vi "AccessData.vi"(0 "Sensitivity1":i32=1, 1 "Sensitivity2":i32=1, 2 "Sensitivity3":i32=1, 3 "Sensitivity4":i32=1, 4 "输入簇":T2, 6 "CH1Enable":bool, 8 "CH2Enable":bool, 10 "CH3Enable":bool, 12 "CH4Enable":bool, 13 "RmOffset":bool, 14 "SamplRate1":T1(ring)=enum."105.468", 15 "SamplRate2":T1(ring)=enum."105.468", 16 "SamplRate3":T1(ring)=enum."105.468", 17 "SamplRate4":T1(ring)=enum."105.468") -> (7 "VibrationWave":dbl[][](array[numeric]) caption="数组", 9 "Speed":u16[](array[numeric]), 11 "Error":bool, 18 "输出簇":T2)   [LabVIEW 2012]
uses:
  <vilib>/measure/madcrms.llb/Basic Averaged DC-RMS for 1 Chan.vi
  <vilib>/measure/NI_MAPro.lvlib
panel:
  out "Humidity_Channel":u8
  out "Temperature_Channel7":u8
  out "Temperature_Channel6":dbl
  out "Temperature_Channel5":dbl
  out "Temperature_Channel4":dbl
  out "Temperature_Channel3":dbl
  out "Temperature_Channel2":dbl
  out "Temperature_Channel1":dbl
  out "系统时间":string
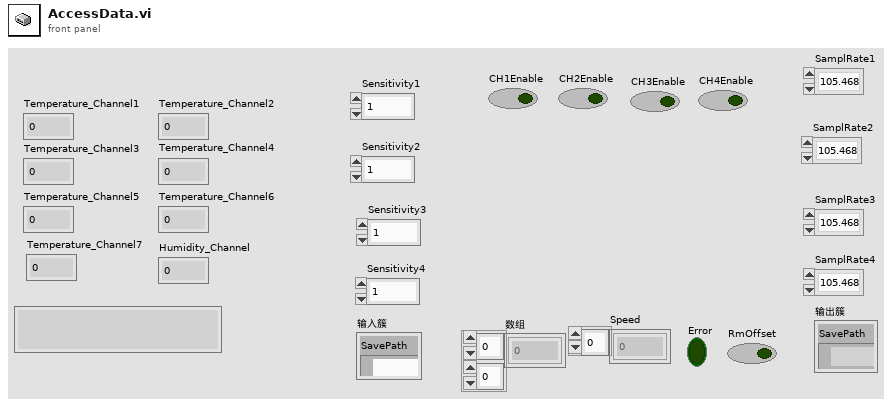
[diagram p1: front panel]
types:
  T1 = enum16{"", "105.468", "52.734", "35.156", "26.367", "21.094", "17.578", "15.067", "13.184", "11.719", "10.545"}
  T2 = cluster{"SavePath":path, "SAVE?":bool, "connection ID":refnum<k5>}
  T3 = enum16{"open", "replace", "create", "open or create", "replace or create", "replace or create with confirmation"}
  T4 = enum16{"big-endian, network order", "native, host order", "little-endian"}
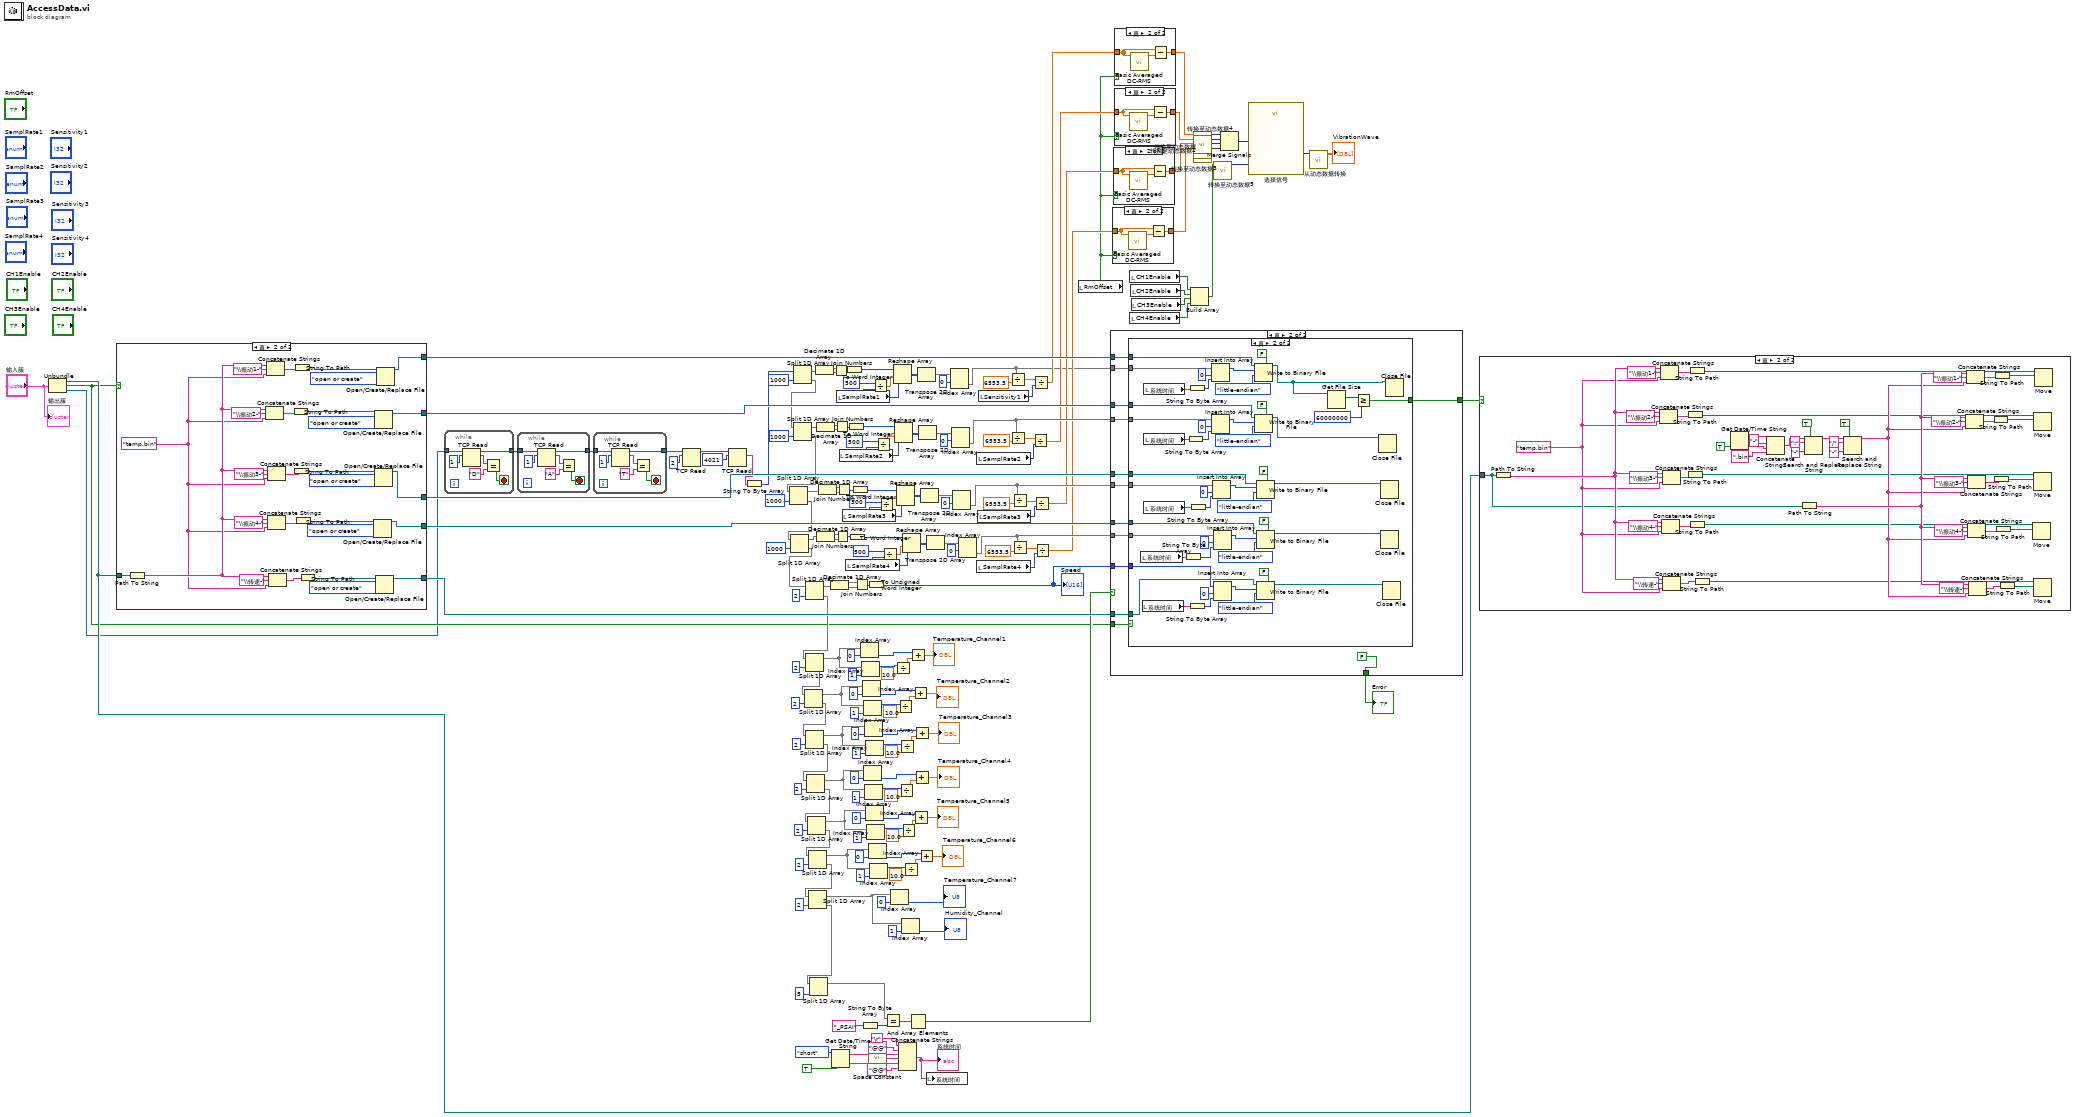
[diagram p0: block diagram]
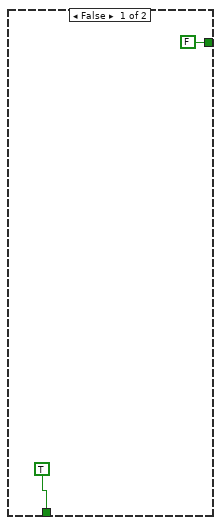
[diagram p6: hidden frame]
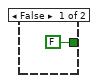
[diagram p7: hidden frame]
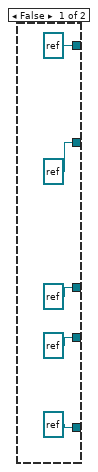
[diagram p8: hidden frame]
diagram:
  n1 = Unbundle("输入簇") -> ("SavePath"=w31:path, "SAVE?"=w30:bool, "connection ID"=w29:refnum<k5>)
  n2 = case shown="真" w30 {
    tunnel: [refnum<file> refnum ("refnum out") w231] -> w198
    tunnel: [refnum<file> refnum ("refnum out") w230] -> w197
    tunnel: [refnum<file> refnum ("refnum out") w229] -> w196
    tunnel: [refnum<file> refnum ("refnum out") w228] -> w195
    tunnel: [refnum<file> refnum ("refnum out") w227] -> w194
    tunnel: w31 -> [_ w204]
    frame False {
    }
    frame True {
      w205 = "temp.bin" ("字符串")
      n3 = Path To String(path=w204) -> (string=w211:string)
      n4 = Concatenate Strings(w211, "\\振动2-" ("字符串"), w205) -> (w218:string)
      n5 = Concatenate Strings(w211, "\\振动1-" ("字符串"), w205) -> (w217:string)
      n6 = Concatenate Strings(w211, "\\振动4-" ("字符串"), w205) -> (w220:string)
      n7 = Concatenate Strings(w211, "\\振动3-" ("字符串"), w205) -> (w219:string)
      n8 = Concatenate Strings(w211, "\\转速-" ("字符串"), w205) -> (w221:string)
      n9 = String To Path(string=w218) -> (path=w215:path)
      n10 = String To Path(string=w219) -> (path=w214:path)
      n11 = String To Path(string=w217) -> (path=w216:path)
      n12 = String To Path(string=w220) -> (path=w213:path)
      n13 = String To Path(string=w221) -> (path=w212:path)
      n14 = Open/Create/Replace File(file path (use dialog)=w213, operation (0:open)=T3."open or create" ("操作(0:open)")) -> (refnum out=w228:refnum<file>)  [unwired: 4 in, 2 out]
      n15 = Open/Create/Replace File(file path (use dialog)=w215, operation (0:open)=T3."open or create" ("操作(0:open)")) -> (refnum out=w230:refnum<file>)  [unwired: 4 in, 2 out]
      n16 = Open/Create/Replace File(file path (use dialog)=w214, operation (0:open)=T3."open or create" ("操作(0:open)")) -> (refnum out=w229:refnum<file>)  [unwired: 4 in, 2 out]
      n17 = Open/Create/Replace File(file path (use dialog)=w212, operation (0:open)=T3."open or create" ("操作(0:open)")) -> (refnum out=w227:refnum<file>)  [unwired: 4 in, 2 out]
      n18 = Open/Create/Replace File(file path (use dialog)=w216, operation (0:open)=T3."open or create" ("操作(0:open)")) -> (refnum out=w231:refnum<file>)  [unwired: 4 in, 2 out]
    }
  }
  n19 = while {
    tunnel: [w234] -> w192
    tunnel: w29 -> [w233]
    stop <- w232 stop-if-true
    n20 = TCP Read(connection ID=w233, bytes to read=1 ("读取的字节")) -> (connection ID out=w234:refnum<k5>, data out=w235:string)  [unwired: 3 in, 1 out]
    n21 = Equal?(x=w235, y="D") -> (x = y?=w232:bool)
  }
  n22 = while {
    tunnel: w192 -> [w243]
    tunnel: [w239] -> w191
    stop <- w238 stop-if-true
    n23 = TCP Read(connection ID=w243, bytes to read=1 ("读取的字节")) -> (connection ID out=w239:refnum<k5>, data out=w242:string)  [unwired: 3 in, 1 out]
    n24 = Equal?(x=w242, y="A") -> (x = y?=w238:bool)
  }
  n25 = while {
    tunnel: w191 -> [w249]
    tunnel: [w245] -> w190
    stop <- w244 stop-if-true
    n26 = TCP Read(connection ID=w249, bytes to read=1 ("读取的字节")) -> (connection ID out=w245:refnum<k5>, data out=w248:string)  [unwired: 3 in, 1 out]
    n27 = Equal?(x=w248, y="T") -> (x = y?=w244:bool)
  }
  n28 = TCP Read(connection ID=w190, bytes to read=2 ("读取的字节")) -> (connection ID out=w63:refnum<k5>)  [unwired: 3 in, 2 out]
  n29 = TCP Read(connection ID=w63, bytes to read=4021 ("最大值(548)")) -> (data out=w174:string)  [unwired: 3 in, 2 out]
  n30 = String To Byte Array(string=w174) -> (unsigned byte array=w173:u8[])
  n31 = Split 1D Array(array=w173, index=1000 ("索引")) -> (first subarray=w103:u8[], second subarray=w100:u8[])
  n32 = Split 1D Array(array=w100, index=1000 ("索引")) -> (first subarray=w99:u8[], second subarray=w96:u8[])
  n33 = Split 1D Array(array=w96, index=1000 ("索引")) -> (first subarray=w95:u8[], second subarray=w94:u8[])
  n34 = Split 1D Array(array=w94, index=1000 ("索引")) -> (first subarray=w91:u8[], second subarray=w104:u8[])
  n35 = Split 1D Array(array=w104, index=2 ("索引")) -> (first subarray=w88:u8[], second subarray=w163:u8[])
  n36 = Split 1D Array(array=w163, index=2 ("索引")) -> (first subarray=w146:u8[], second subarray=w162:u8[])
  n37 = Split 1D Array(array=w162, index=2 ("索引")) -> (first subarray=w110:u8[], second subarray=w161:u8[])
  n38 = Split 1D Array(array=w161, index=2 ("索引")) -> (first subarray=w109:u8[], second subarray=w148:u8[])
  n39 = Split 1D Array(array=w148, index=2 ("索引")) -> (first subarray=w108:u8[], second subarray=w157:u8[])
  n40 = Split 1D Array(array=w157, index=2 ("索引")) -> (first subarray=w107:u8[], second subarray=w156:u8[])
  n41 = Split 1D Array(array=w156, index=2 ("索引")) -> (first subarray=w106:u8[], second subarray=w147:u8[])
  n42 = Split 1D Array(array=w147, index=2 ("索引")) -> (first subarray=w105:u8[], second subarray=w83:u8[])
  n43 = Split 1D Array(array=w83, index=5 ("索引")) -> (first subarray=w82:u8[])  [unwired: 1 out]
  n44 = Decimate 1D Array(w103) -> (w102:u8[], w101:u8[])
  n45 = Decimate 1D Array(w91) -> (w90:u8[], w89:u8[])
  n46 = Decimate 1D Array(w99) -> (w98:u8[], w97:u8[])
  n47 = Decimate 1D Array(w95) -> (w93:u8[], w92:u8[])
  n48 = Decimate 1D Array(w88) -> (w87:u8[], w86:u8[])
  n49 = Get Date/Time String(date format (0)=enum16{"short", "long", "abbreviated"}."short" ("日期格式(0)"), want seconds? (F)=TRUE ("需要秒？(F)")) -> (date string=w170:string, time string=w164:string)  [unwired: 1 in]
  n50 = Join Numbers(hi=w102, lo=w101) -> ((hi.lo)=w186:u16[])
  n51 = Join Numbers(hi=w98, lo=w97) -> ((hi.lo)=w181:u16[])
  n52 = Join Numbers(hi=w90, lo=w89) -> ((hi.lo)=w183:u16[])
  n53 = Join Numbers(hi=w93, lo=w92) -> ((hi.lo)=w182:u16[])
  n54 = local read "SamplRate1"() -> (w42:T1)
  n55 = local read "SamplRate2"() -> (w38:T1)
  n56 = local read "SamplRate3"() -> (w37:T1)
  n57 = To Word Integer(number=w186) -> (16bit integer=w3:i16[])
  n58 = local read "SamplRate4"() -> (w33:T1)
  n59 = To Word Integer(number=w181) -> (16bit integer=w50:i16[])
  n60 = To Word Integer(number=w183) -> (16bit integer=w48:i16[])
  n61 = To Word Integer(number=w182) -> (16bit integer=w49:i16[])
  n62 = Join Numbers(hi=w87, lo=w86) -> ((hi.lo)=w85:u16[])
  n63 = Index Array(array=w146, index=0 ("索引")) -> (element=w141:u8)
  n64 = Index Array(array=w146, index=1 ("索引")) -> (element=w143:u8)
  n65 = String To Byte Array(string="_PSAI") -> (unsigned byte array=w177:u8[])
  n66 = Index Array(array=w110, index=0 ("索引")) -> (element=w135:u8)
  n67 = Index Array(array=w110, index=1 ("索引")) -> (element=w137:u8)
  n68 = Index Array(array=w108, index=0 ("索引")) -> (element=w123:u8)
  n69 = Index Array(array=w109, index=0 ("索引")) -> (element=w129:u8)
  n70 = Index Array(array=w108, index=1 ("索引")) -> (element=w125:u8)
  n71 = Index Array(array=w109, index=1 ("索引")) -> (element=w131:u8)
  n72 = Index Array(array=w107, index=0 ("索引")) -> (element=w117:u8)
  n73 = Index Array(array=w107, index=1 ("索引")) -> (element=w119:u8)
  n74 = To Unsigned Word Integer(number=w85) -> (unsigned 16bit integer=w81:u16[])
  "Speed" <- w81
  n75 = Index Array(array=w106, index=0 ("索引")) -> (element=w111:u8)
  n76 = call <vilib>:"Space Constant.vi"() -> ("String"=w166:string)
  n77 = Index Array(array=w106, index=1 ("索引")) -> (element=w113:u8)
  n78 = Divide(x=500, y=w42) -> (x/y=w43:dbl)
  n79 = Divide(x=500, y=w38) -> (x/y=w39:dbl)
  n80 = Divide(x=500, y=w37) -> (x/y=w36:dbl)
  n81 = Divide(x=500, y=w33) -> (x/y=w35:dbl)
  n82 = Equal?(x=w82, y=w177) -> (x = y?=w176:bool[])
  n83 = Index Array(array=w105, index=0 ("索引")) -> (element=→"Temperature_Channel7":u8)
  n84 = Reshape Array(w3, w43, w42) -> (w61:i16[][])
  n85 = Divide(x=w143, y=10.0) -> (x/y=w142:dbl)
  n86 = Reshape Array(w50, w39, w38) -> (w58:i16[][])
  n87 = Reshape Array(w49, w36, w37) -> (w55:i16[][])
  n88 = Divide(x=w137, y=10.0) -> (x/y=w136:dbl)
  n89 = Divide(x=w125, y=10.0) -> (x/y=w124:dbl)
  n90 = Divide(x=w131, y=10.0) -> (x/y=w130:dbl)
  n91 = Concatenate Strings("\r", "@@" ("字符串"), w170, w166, w164, "@@" ("字符串")) -> (w169:string)
  "系统时间" <- w169
  n92 = Divide(x=w119, y=10.0) -> (x/y=w118:dbl)
  n93 = Index Array(array=w105, index=1 ("索引")) -> (element=→"Humidity_Channel":u8)
  n94 = Reshape Array(w48, w35, w33) -> (w52:i16[][])
  n95 = Divide(x=w113, y=10.0) -> (x/y=w112:dbl)
  n96 = And Array Elements(Boolean array=w176) -> (logical AND=w175:bool)
  n97 = Add(x=w141, y=w142) -> (x+y=→"Temperature_Channel1":dbl)
  n98 = Add(x=w135, y=w136) -> (x+y=→"Temperature_Channel2":dbl)
  n99 = Add(x=w117, y=w118) -> (x+y=→"Temperature_Channel5":dbl)
  n100 = Add(x=w123, y=w124) -> (x+y=→"Temperature_Channel4":dbl)
  n101 = Add(x=w129, y=w130) -> (x+y=→"Temperature_Channel3":dbl)
  n102 = Transpose 2D Array(2D array=w61) -> (transposed array=w60:i16[][])
  n103 = Add(x=w111, y=w112) -> (x+y=→"Temperature_Channel6":dbl)
  n104 = Transpose 2D Array(2D array=w58) -> (transposed array=w57:i16[][])
  n105 = Transpose 2D Array(2D array=w55) -> (transposed array=w54:i16[][])
  n106 = Transpose 2D Array(2D array=w52) -> (transposed array=w51:i16[][])
  n107 = local write "系统时间"(w169) -> ()
  n108 = Index Array(array=w60, index (row)=0 ("索引 (行)")) -> (element=w4:i16[])  [unwired: 1 in]
  n109 = Index Array(array=w57, index (row)=0 ("索引 (行)")) -> (element=w47:i16[])  [unwired: 1 in]
  n110 = Index Array(array=w54, index (row)=0 ("索引 (行)")) -> (element=w46:i16[])  [unwired: 1 in]
  n111 = Index Array(array=w51, index (row)=0 ("索引 (行)")) -> (element=w45:i16[])  [unwired: 1 in]
  n112 = local read "SamplRate2"() -> (w27:T1)
  n113 = local read "SamplRate4"() -> (w25:T1)
  n114 = local read "SamplRate3"() -> (w26:T1)
  n115 = local read "Sensitivity1"() -> (w28:i32)
  n116 = Divide(x=w4, y=6553.5) -> (x/y=w73:dbl[])
  n117 = Divide(x=w47, y=6553.5) -> (x/y=w74:dbl[])
  n118 = Divide(x=w46, y=6553.5) -> (x/y=w75:dbl[])
  n119 = Divide(x=w45, y=6553.5) -> (x/y=w76:dbl[])
  n120 = Divide(x=w74, y=w27) -> (x/y=w24:dbl[])
  n121 = Divide(x=w73, y=w28) -> (x/y=w7:dbl[])
  n122 = Divide(x=w75, y=w26) -> (x/y=w23:dbl[])
  n123 = Divide(x=w76, y=w25) -> (x/y=w22:dbl[])
  n124 = local read "RmOffset"() -> (w21:bool)
  n125 = case shown="真" w175 {
    tunnel: [TRUE FALSE] -> w64
    tunnel: w4 -> [_ w264]
    tunnel: w47 -> [_ w263]
    tunnel: w46 -> [_ w262]
    tunnel: w45 -> [_ w261]
    tunnel: w81 -> [_ w260]
    tunnel: w198 -> [_ w258]
    tunnel: w197 -> [_ w257]
    tunnel: w196 -> [_ w256]
    tunnel: w195 -> [_ w255]
    tunnel: w194 -> [_ w254]
    tunnel: w30 -> [_ w253]
    tunnel: [FALSE w252] -> w193
    frame False {
    }
    frame True {
      n126 = case shown="真" w253 {
        tunnel: w264 -> [_ w312]
        tunnel: w263 -> [_ w292]
        tunnel: w262 -> [_ w291]
        tunnel: w261 -> [_ w290]
        tunnel: w260 -> [_ w289]
        tunnel: w258 -> [_ w278]
        tunnel: w257 -> [_ w277]
        tunnel: w256 -> [_ w276]
        tunnel: w255 -> [_ w275]
        tunnel: w254 -> [_ w274]
        tunnel: [FALSE w271] -> w252
        frame False {
        }
        frame True {
          n127 = local read "系统时间"() -> (w286:string)
          n128 = local read "系统时间"() -> (w288:string)
          n129 = local read "系统时间"() -> (w280:string)
          n130 = local read "系统时间"() -> (w282:string)
          n131 = local read "系统时间"() -> (w284:string)
          n132 = String To Byte Array(string=w286) -> (unsigned byte array=w285:u8[])
          n133 = String To Byte Array(string=w282) -> (unsigned byte array=w281:u8[])
          n134 = String To Byte Array(string=w280) -> (unsigned byte array=w279:u8[])
          n135 = String To Byte Array(string=w288) -> (unsigned byte array=w287:u8[])
          n136 = String To Byte Array(string=w284) -> (unsigned byte array=w283:u8[])
          n137 = Insert Into Array(array=w312, index=0 ("索引"), new element=w279) -> (w310:i16[])
          n138 = Insert Into Array(array=w292, index=0 ("索引"), new element=w281) -> (w306:i16[])
          n139 = Insert Into Array(array=w291, index=0 ("索引"), new element=w283) -> (w302:i16[])
          n140 = Insert Into Array(array=w290, index=0 ("索引"), new element=w285) -> (w298:i16[])
          n141 = Insert Into Array(array=w289, index=0 ("索引"), new element=w287) -> (w294:u16[])
          n142 = Write to Binary File(file (use dialog)=w278, data=w310, 5:FALSE ("预置数组或字符串大小？(T)"), 9:T4."little-endian" ("字节顺序(0:big-endian, network order)")) -> (refnum out=w270:refnum<file>)  [unwired: 2 in, 2 out]
          n143 = Write to Binary File(file (use dialog)=w277, data=w306, 5:FALSE ("预置数组或字符串大小？(T)"), 9:T4."little-endian" ("字节顺序(0:big-endian, network order)")) -> (refnum out=w269:refnum<file>)  [unwired: 2 in, 2 out]
          n144 = Write to Binary File(file (use dialog)=w276, data=w302, 5:FALSE ("预置数组或字符串大小？(T)"), 9:T4."little-endian" ("字节顺序(0:big-endian, network order)")) -> (refnum out=w268:refnum<file>)  [unwired: 2 in, 2 out]
          n145 = Write to Binary File(file (use dialog)=w275, data=w298, 5:FALSE ("预置数组或字符串大小？(T)"), 9:T4."little-endian" ("字节顺序(0:big-endian, network order)")) -> (refnum out=w267:refnum<file>)  [unwired: 2 in, 2 out]
          n146 = Write to Binary File(file (use dialog)=w274, data=w294, 5:FALSE ("预置数组或字符串大小？(T)"), 9:T4."little-endian" ("字节顺序(0:big-endian, network order)")) -> (refnum out=w266:refnum<file>)  [unwired: 2 in, 2 out]
          n147 = Get File Size(file=w270) -> (size (in bytes)=w273:i64)  [unwired: 1 in, 2 out]
          n148 = Greater Or Equal?(x=w273, y=i64 60000000) -> (x >= y?=w271:bool)
          n149 = Close File(refnum=w269) -> ()  [unwired: 1 in, 2 out]
          n150 = Close File(refnum=w268) -> ()  [unwired: 1 in, 2 out]
          n151 = Close File(refnum=w267) -> ()  [unwired: 1 in, 2 out]
          n152 = Close File(refnum=w266) -> ()  [unwired: 1 in, 2 out]
          n153 = Close File(refnum=w270) -> ()  [unwired: 1 in, 2 out]
        }
      }
    }
  }
  "Error" <- w64
  n154 = case shown="真" w21 {
    tunnel: w22 -> [w314 w315]
    tunnel: [w314 w316] -> w10
    frame False {
    }
    frame True {
      n155 = call-poly <vilib>:"Basic Averaged DC-RMS.vi"("signal in"=w315) -> ("DC value"=w317:dbl)  [unwired: 7 in, 3 out]
      n156 = Subtract(x=w315, y=w317) -> (x-y=w316:dbl[])
    }
  }
  n157 = case shown="真" w21 {
    tunnel: w23 -> [w318 w319]
    tunnel: [w318 w320] -> w12
    frame False {
    }
    frame True {
      n158 = call-poly <vilib>:"Basic Averaged DC-RMS.vi"("signal in"=w319) -> ("DC value"=w321:dbl)  [unwired: 7 in, 3 out]
      n159 = Subtract(x=w319, y=w321) -> (x-y=w320:dbl[])
    }
  }
  n160 = case shown="真" w21 {
    tunnel: w24 -> [w322 w323]
    tunnel: [w322 w324] -> w14
    frame False {
    }
    frame True {
      n161 = call-poly <vilib>:"Basic Averaged DC-RMS.vi"("signal in"=w323) -> ("DC value"=w325:dbl)  [unwired: 7 in, 3 out]
      n162 = Subtract(x=w323, y=w325) -> (x-y=w324:dbl[])
    }
  }
  n163 = case shown="真" w21 {
    tunnel: w7 -> [w326 w327]
    tunnel: [w326 w328] -> w6
    frame False {
    }
    frame True {
      n164 = call-poly <vilib>:"Basic Averaged DC-RMS.vi"("signal in"=w327) -> ("DC value"=w329:dbl)  [unwired: 7 in, 3 out]
      n165 = Subtract(x=w327, y=w329) -> (x-y=w328:dbl[])
    }
  }
  n166 = local read "CH1Enable"() -> (w16:bool)
  n167 = local read "CH4Enable"() -> (w17:bool)
  n168 = local read "CH2Enable"() -> (w19:bool)
  n169 = local read "CH3Enable"() -> (w18:bool)
  n170 = Build Array(w16, w19, w18, w17) -> (w15:bool[])
  n171 = call "转换至动态数据4"("Array"=w6) -> ("Dynamic Data Type"=w8:dynamicdata)  [unwired: 3 in]
  n172 = call "转换至动态数据"("Array"=w14) -> ("Dynamic Data Type"=w13:dynamicdata)  [unwired: 3 in]
  n173 = call "转换至动态数据2"("Array"=w12) -> ("Dynamic Data Type"=w11:dynamicdata)  [unwired: 3 in]
  n174 = call "转换至动态数据3"("Array"=w10) -> ("Dynamic Data Type"=w9:dynamicdata)  [unwired: 3 in]
  n175 = call "转换至动态数据5"("Array"=w15) -> ("Dynamic Data Type"=w20:dynamicdata)  [unwired: 3 in]
  n176 = Merge Signals(w8, w13, w11, w9) -> (w5:dynamicdata)
  n177 = call "选择信号"("Selector Input"=w20, "Signals"=w5) -> ("Signal Out"=w2:dynamicdata)  [unwired: 8 in, 1 out]
  n178 = call "从动态数据转换"("Dynamic Data Type"=w2) -> ("Array"=→"VibrationWave":dbl[][])  [unwired: 3 in]
  n179 = case shown="真" w193 {
    tunnel: w31 -> [_ w330]
    frame False {
    }
    frame True {
      w341 = "temp.bin" ("字符串")
      n180 = Path To String(path=w330) -> (string=w347:string)
      n181 = Concatenate Strings(w347, "\\振动2-" ("字符串"), w341) -> (w349:string)
      n182 = Concatenate Strings(w347, "\\振动1-" ("字符串"), w341) -> (w348:string)
      n183 = Concatenate Strings(w347, "\\振动4-" ("字符串"), w341) -> (w351:string)
      n184 = Concatenate Strings(w347, "\\振动3-" ("字符串"), w341) -> (w350:string)
      n185 = Concatenate Strings(w347, "\\转速-" ("字符串"), w341) -> (w352:string)
      n186 = String To Path(string=w349) -> (path=w338:path)
      n187 = String To Path(string=w350) -> (path=w337:path)
      n188 = String To Path(string=w348) -> (path=w340:path)
      n189 = String To Path(string=w351) -> (path=w336:path)
      n190 = String To Path(string=w352) -> (path=w335:path)
      n191 = Get Date/Time String(want seconds? (F)=TRUE ("需要秒？(F)")) -> (date string=w365:string, time string=w362:string)  [unwired: 2 in]
      n192 = Concatenate Strings(w365, "-" ("字符串"), w362, ".bin" ("字符串")) -> (w361:string)
      n193 = Path To String(path=w330) -> (string=w372:string)
      n194 = Search and Replace String(replace all?=TRUE ("替换全部？(F)"), input string=w361, search string=":" ("搜索字符串"), replace string="-" ("替换字符串(\"\")")) -> (result string=w354:string)  [unwired: 4 in, 3 out]
      n195 = Search and Replace String(replace all?=TRUE ("替换全部？(F)"), input string=w354, search string="/" ("搜索字符串"), replace string="-" ("替换字符串(\"\")")) -> (result string=w353:string)  [unwired: 4 in, 3 out]
      n196 = Concatenate Strings(w372, "\\振动2-" ("字符串"), w353) -> (w374:string)
      n197 = Concatenate Strings(w372, "\\振动1-" ("字符串"), w353) -> (w373:string)
      n198 = Concatenate Strings(w372, "\\振动4-" ("字符串"), w353) -> (w376:string)
      n199 = Concatenate Strings(w372, "\\振动3-" ("字符串"), w353) -> (w375:string)
      n200 = Concatenate Strings(w372, "\\转速-" ("字符串"), w353) -> (w377:string)
      n201 = String To Path(string=w374) -> (path=w334:path)
      n202 = String To Path(string=w375) -> (path=w333:path)
      n203 = String To Path(string=w373) -> (path=w339:path)
      n204 = String To Path(string=w376) -> (path=w332:path)
      n205 = String To Path(string=w377) -> (path=w331:path)
      n206 = Move(source path=w336, 10:w332) -> ()  [unwired: 3 in, 3 out]
      n207 = Move(source path=w338, 10:w334) -> ()  [unwired: 3 in, 3 out]
      n208 = Move(source path=w337, 10:w333) -> ()  [unwired: 3 in, 3 out]
      n209 = Move(source path=w335, 10:w331) -> ()  [unwired: 3 in, 3 out]
      n210 = Move(source path=w340, 10:w339) -> ()  [unwired: 3 in, 3 out]
    }
  }
  "输出簇" <- "输入簇"
